vi "FPGA Resampling.vi"   [LabVIEW 2014, in "NI_EP_Resample_FPGA.lvlib"]
doc: "Resamples even-time-spaced voltage and current signals into even-angle-spaced signals. The input signals must have a sample rate of 50 kHz. The output signals are synchronous with the line frequency with a constant number of samples per cycle. Use the Resampling for Power Quality VI if you want to perform resampling on the host computer. You must manually select the polymorphic instance to use.\n\nThis VI supports measuring single-bus single-line and single-bus multiple-line systems."
uses:
  <vilib>/addons/Electrical Power/PQ/Resampling/NI_EP_Resample_FPGA.lvlib
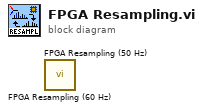
[diagram p0: block diagram]
diagram:
  n1 = call <vilib>:"FPGA Resampling (60 Hz).vi"() -> ()  [unwired: 12 in, 4 out]
  n2 = call <vilib>:"FPGA Resampling (50 Hz).vi"() -> ()  [unwired: 12 in, 4 out]
